vi "Open Producer Tag Cluster.vi"(8 "error in":errorcluster, 9 "Create if not found? (T)":bool=TRUE, 10 "Cluster":variant, 11 "Channel Name":string) -> (0 "error out":errorcluster, 3 "ADAS HIL Channel":refnum<k21>)   [LabVIEW 2023, in "Utilities.lvlib"]
uses:
  Utilities.lvlib
  826f5016-74ba-49aa-9f0b-5b6dae313aec.vi
  AdasHilServices.dll
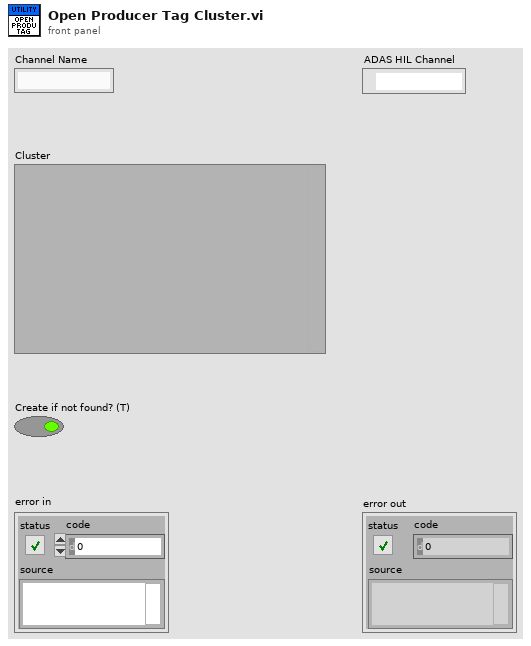
[diagram p1: front panel]
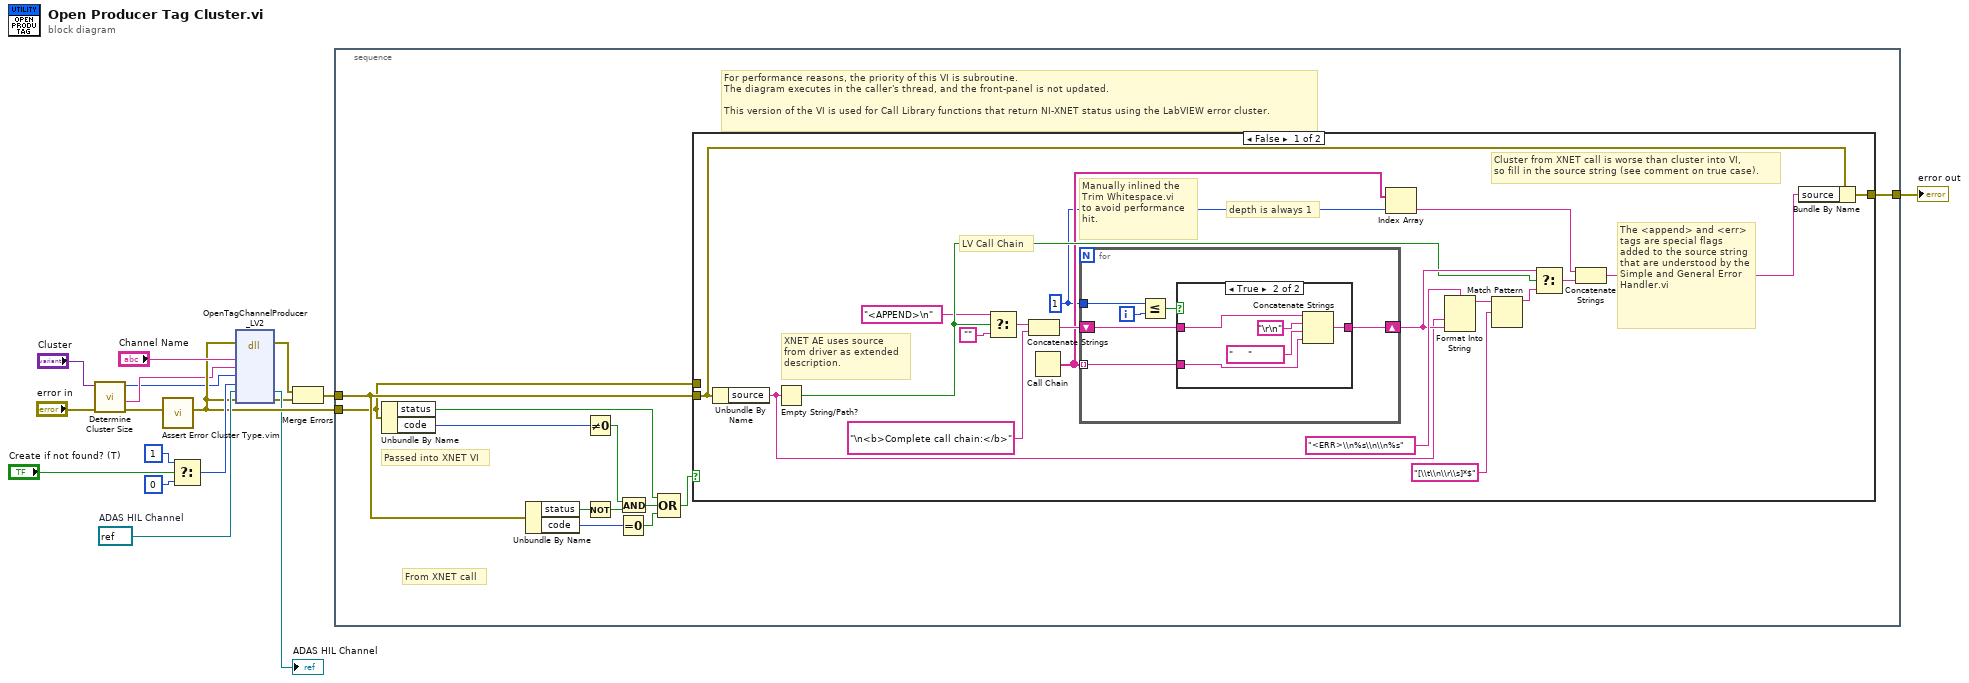
[diagram p0: block diagram]
diagram:
  w9 = refnum<k21> refnum  # ADAS HIL Channel
  n1 = call "Determine Cluster Size.vi"("error in"="error in", "Variant"="Cluster") -> ("error out"=w4:errorcluster, "Title"=w3:string, "Total Size"=w2:i32)  [unwired: 3 in, 4 out]
  n2 = call "Assert Error Cluster Type.vim"("value in"=w4) -> ("value out"=w8:errorcluster)  [unwired: 8 in]
  n3 = Select(t=u32 1, s="Create if not found? (T)", f=u32 0 ("t")) -> (s? t:f=w10:u32)
  n4 = dll-call lib="AdasHilServices.*" fn="OpenTagChannelProducer_LV2"(error in=w8, "channelName"="Channel Name", "channelTypeDescription"=w3, "elementSize"=w2, "flags"=w10, "handleOut"=w9, "error"=w8) -> (error out=w12:errorcluster, "handleOut"=→"ADAS HIL Channel":refnum<k21>, "error"=w6:errorcluster)  [unwired: 7 in, 1 out]
  n5 = Merge Errors(w12, w6) -> (w14:errorcluster)
  n6 = stacked-sequence {
    tunnel: w14 -> [w23]
    tunnel: w8 -> [w19]
    tunnel: [w18] -> w13
    frame #0 {
      # "From XNET call"
      # "Passed into XNET VI"
      # "For performance reasons, the priority of this VI is subroutine.\nThe diagram executes in the caller's thread, and the front-panel is not updated.\n\nThis version of the VI is used for Call Library functions that return NI-XNET status using the LabVIEW error cluster."
      n7 = Unbundle By Name(w19) -> ("status"=w21:bool, "code"=w22:i32)
      n8 = Unbundle By Name(w23) -> ("status"=w26:bool, "code"=w28:i32)
      n9 = Not Equal To 0?(x=w22) -> (x != 0?=w25:bool)
      n10 = Not(x=w26) -> (.not. x?=w27:bool)
      n11 = Equal To 0?(x=w28) -> (x = 0?=w29:bool)
      n12 = And(x=w25, y=w27) -> (x .and. y?=w24:bool)
      n13 = Compound Arithmetic op=OR(w21, w24, w29) -> (w20:bool)
      n14 = case shown="False" w20 {
        tunnel: [w48 w61] -> w18
        tunnel: w19 -> [_ w61]
        tunnel: w23 -> [w31 _]
        frame False {
          w32 = 1 ("depth (1)")
          # "LV Call Chain"
          # "XNET AE uses source\nfrom driver as extended\ndescription."
          # "Cluster from XNET call is worse than cluster into VI,\nso fill in the source string (see comment on true case)."
          # "depth is always 1"
          # "Manually inlined the\nTrim Whitespace.vi\nto avoid performance\nhit."
          # "The <append> and <err> tags are special flags added to the source string that are understood by the Simple and General Error Handler.vi"
          n15 = Unbundle By Name(w31) -> ("source"=w30:string)
          n16 = Empty String/Path?(string/path=w30) -> (empty?=w43:bool)
          n17 = Select(t="<APPEND>\n", s=w43, f="") -> (s? t:f=w34:string)
          n18 = Concatenate Strings(w34, "\n<b>Complete call chain:</b>" ("call chain header")) -> (w37:string)
          n19 = Call Chain() -> (call chain=w33:string[])
          n20 = for {
            tunnel: w33 -> [w52] mode=indexing
            shift-right: [w54] -> w45
            shift-left: w37 -> [w53]
            tunnel: w32 -> [w49]
            i -> [w50]
            n21 = Less Or Equal?(x=w49, y=w50) -> (x <= y?=w51:bool)
            n22 = case shown="True" w51 {
              tunnel: [w55 w60] -> w54
              tunnel: w53 -> [w55 w58]
              tunnel: w52 -> [_ w57]
              frame False {
              }
              frame True {
                n23 = Concatenate Strings(w58, "\r\n", "     ", w57) -> (w60:string)
              }
            }
          }
          n24 = Index Array(array=w33, index=w32) -> (element=w39:string)
          n25 = Format Into String(format string="<ERR>\\n%s\\n\\n%s", w30, w45) -> (resulting string=w41:string)  [unwired: 2 in, 1 out]
          n26 = Match Pattern(string=w41, regular expression="[\\t\\n\\r\\s]*$") -> (before substring=w40:string)  [unwired: 1 in, 3 out]
          n27 = Select(t=w45, s=w43, f=w40) -> (s? t:f=w44:string)
          n28 = Concatenate Strings(w39, w44) -> (w47:string)
          n29 = Bundle By Name(cluster=w31, "source"=w47) -> (w48:errorcluster)
        }
        frame True {
          # "Cluster from XNET call is not worse than cluster into VI,\nso do nothing.\n\nError is status==T.\nWarning is status==F code!=0.\nSuccess is status==F code==0.\n\nError is worse than Warning.\nWarning is worse than Success"
        }
      }
    }
  }
  "error out" <- w13
